vi "ST - Stop motion.vi"(8 "error in":errorcluster, 10 "Axis":i8=1 min=1 max=6 step=1, 11 "Address / Port":i16=1 min=1 max=31 step=1) -> (0 "error out":errorcluster, 2 "Axis dup":i8=1 min=1 max=6 step=1, 3 "Address / Port dup":i16=1 min=1 max=31 step=1)   [LabVIEW 2014]
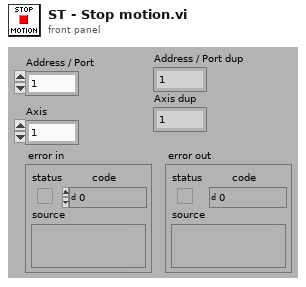
[diagram p1: front panel]
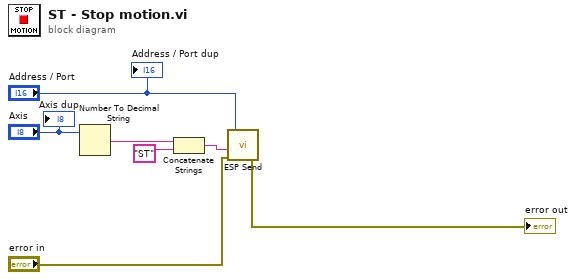
[diagram p0: block diagram]
diagram:
  n1 = Number To Decimal String(number="Axis") -> (decimal integer string=w6:string)  [unwired: 1 in]
  n2 = Concatenate Strings(w6, "ST" ("Substring")) -> (w4:string)
  n3 = call "ESP Send.vi"("error in"="error in", "Command String"=w4, "Address / Port"="Address / Port") -> ("error out"=→"error out":errorcluster)  [unwired: 3 in, 1 out]
  "Address / Port dup" <- "Address / Port"
  "Axis dup" <- "Axis"
